vi "PROJETO_PAINEL_INSTRUMENTOS.vi"() -> ()   [LabVIEW 2018]
panel:
  in  "OFF\n\n\nON":bool
  out "Reduzir mudança":bool
  in  "Gear":dbl=1.0 min=1.0 max=6.0 step=1.0
  out "Temperatura":bool
  out "Pressão":bool
  out "Subir mudança":bool
  out "RPM":dbl(knob) scale=0.0..10000.0
  out "Pressão":dbl(knob) scale=0.0..20.0
  out "Temperatura":dbl(knob) scale=0.0..300.0
  out "Velocímetro":dbl(knob) scale=0.0..200.0
  in  "Acelerador":dbl(slide) scale=0.0..200.0
  # "Inputs de temperatura e pressão simulados por números aleatórios"
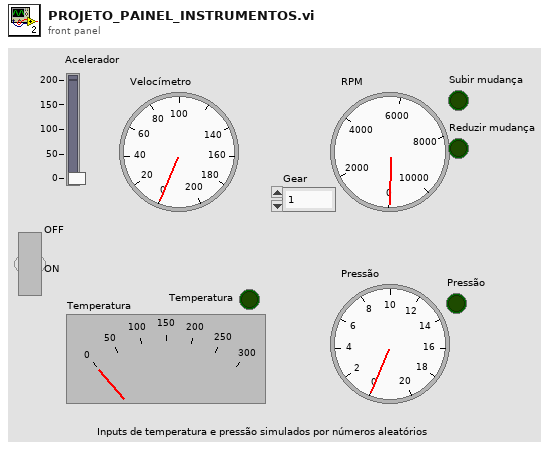
[diagram p1: front panel]
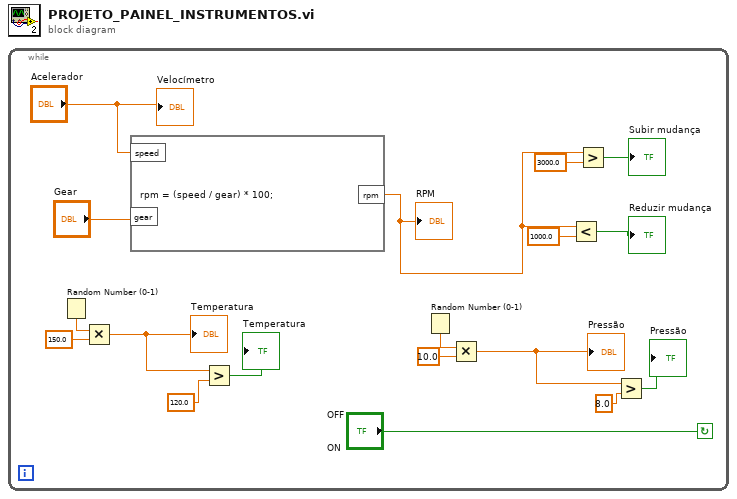
[diagram p0: block diagram]
diagram:
  n1 = while {
    stop <- "OFF\n\n\nON" continue-if-true
    n2 = Random Number (0-1)() -> (number: 0 to 1=w9:dbl)
    n3 = Multiply(x=w9, y=150.0) -> (x*y=w10:dbl)
    "Temperatura" <- w10
    n4 = formula code="rpm = (speed / gear) * 100;"("speed"="Acelerador", "gear"="Gear") -> ("rpm"=w13:dbl)
    "RPM" <- w13
    n5 = Greater?(x=w10, y=120.0) -> (0:→"Temperatura":bool)
    n6 = Random Number (0-1)() -> (number: 0 to 1=w7:dbl)
    n7 = Multiply(x=w7, y=10.0) -> (x*y=w2:dbl)
    "Pressão" <- w2
    n8 = Less?(x=w13, y=1000.0) -> (x < y?=→"Reduzir mudança":bool)
    n9 = Greater?(x=w13, y=3000.0) -> (0:→"Subir mudança":bool)
    n10 = Greater?(x=w2, y=8.0) -> (0:→"Pressão":bool)
    "Velocímetro" <- "Acelerador"
  }
